vi "Dynamic Launch Nested Actor.vi"(8 "error in (no error)":errorcluster, 11 "UI ActorTop in":refnum<class "CallActorCenter.lvclass">) -> (0 "error out":errorcluster, 3 "UI ActorTop out":refnum<class "CallActorCenter.lvclass">)   [LabVIEW 2021, in "CallActorCenter.lvclass"]
doc: "Use Launch Nested Actor.vi to dynamic load child VI.\n2015-04-02 12:54:56\n蒋松\njiangsong@outlook.com"
uses:
  CallActorCenter.lvclass
  C:/Program Files (x86)/National Instruments/LabVIEW 2021/vi.lib/ActorFramework/Actor/Actor.lvclass
  C:/Program Files (x86)/National Instruments/LabVIEW 2021/user.lib/John_Lib/AbstractActorTemplate/AbstractActorTemplate/UIActorTop.lvclass
  CallActorCenter.lvclass/CallActorCenter.ctl
  <vilib>/ActorFramework/Message Enqueuer/Message Enqueuer.lvclass
  <userlib>/John_Lib/AbstractActorTemplate/AbstractActorTemplate/UIActorTop.lvclass
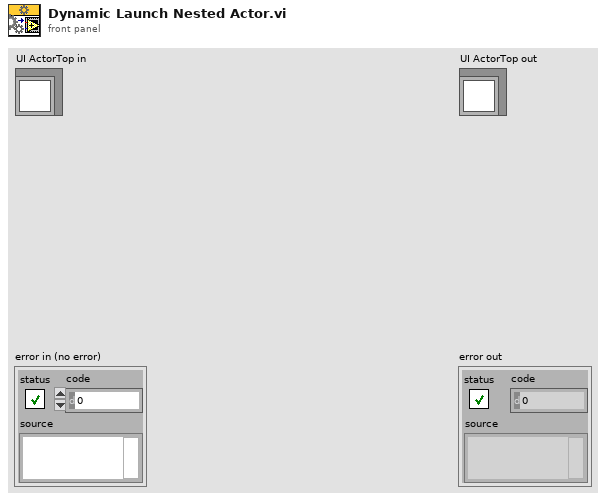
[diagram p1: front panel]
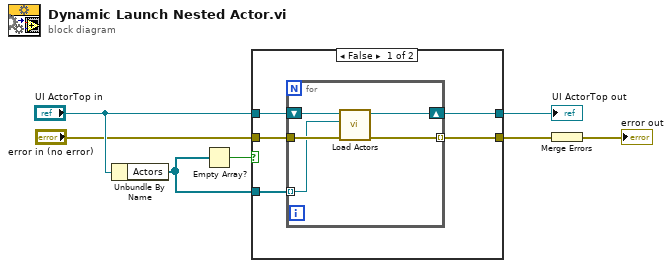
[diagram p0: block diagram]
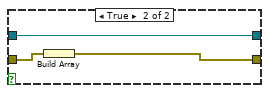
[diagram p2: hidden frame]
diagram:
  n1 = Unbundle By Name("UI ActorTop in") -> ("Actors"=w6:refnum<class "UIActorTop.lvclass">[])
  n2 = Empty Array?(array=w6) -> (empty?=w7:bool)
  n3 = case shown="False" w7 {
    tunnel: "error in (no error)" -> [w12 w19]
    tunnel: "UI ActorTop in" -> [w11 w20]
    tunnel: [w10 w20] -> w1
    tunnel: [w9 w18] -> w5
    tunnel: w6 -> [w8 _]
    frame False {
      n4 = for {
        tunnel: w8 -> [w14] mode=indexing
        tunnel: w12 -> [w15]
        shift-right: [w16] -> w10
        shift-left: w11 -> [w17]
        tunnel: [w13] -> w9 mode=indexing
        n5 = call <userlib>:"Load Actors.vi"("error in (no error)"=w15, "NestedActor"=w14, "UIActorTop in"=w17) -> ("error out"=w13:errorcluster, "UIActorTop out"=w16:refnum<class "CallActorCenter.lvclass">)  [unwired: 7 in]
      }
    }
    frame True {
      n6 = Build Array(w19) -> (w18:errorcluster[])
    }
  }
  "UI ActorTop out" <- w1
  n7 = Merge Errors(w5) -> (→"error out":errorcluster)
